vi "Collect and Set PWM.vi"(11 "Aircraft ID":u8) -> (3 "output cluster":T1)   [LabVIEW 2014]
uses:
  Aircraft Information/Sub VI/Get Aircraft RC Override.vi
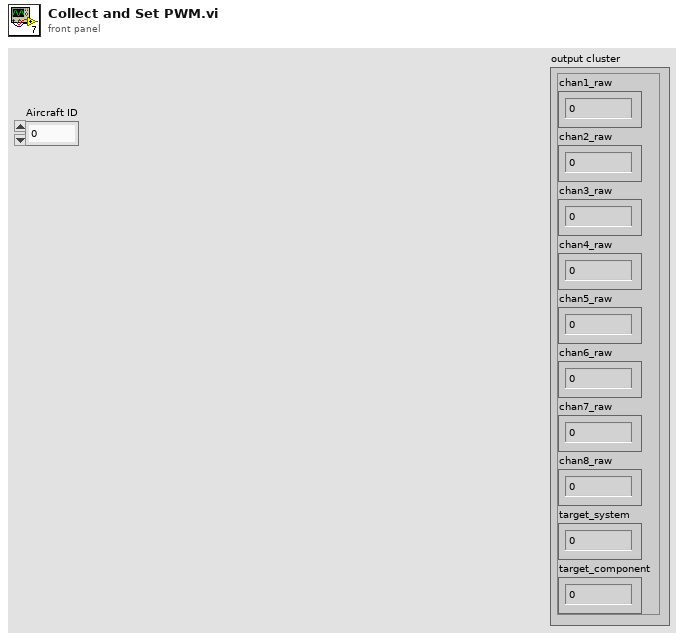
[diagram p1: front panel]
types:
  T1 = cluster{"chan1_raw":u16, "chan2_raw":u16, "chan3_raw":u16, "chan4_raw":u16, "chan5_raw":u16, "chan6_raw":u16, "chan7_raw":u16, "chan8_raw":u16, "target_system":u8, "target_component":u8}
  T2 = typedef "RC Override.ctl" = cluster{"Throttle":u16, "Roll":u16, "Pitch":u16, "Yaw":u16, "Arm":bool, "Disarm":bool, "Aircraft Mode":T3}
  T3 = typedef "Aircraft Mode.ctl" = enum16{"Loiter", "Stabalise", "Failsafe", "Emergency Stop"}
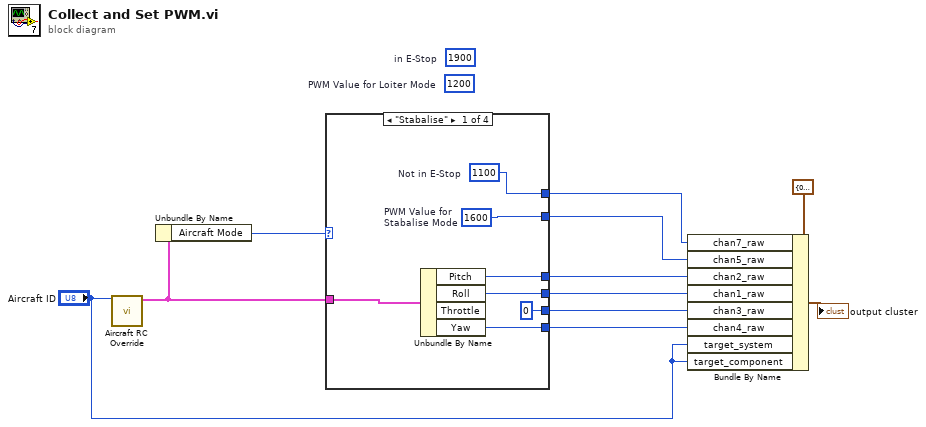
[diagram p0: block diagram]
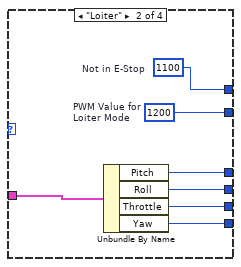
[diagram p2: hidden frame]
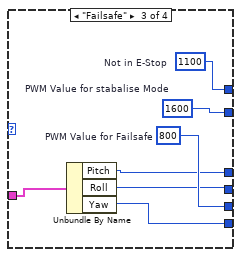
[diagram p3: hidden frame]
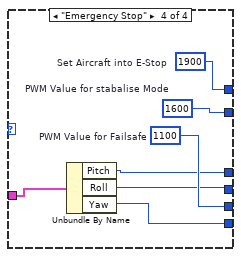
[diagram p4: hidden frame]
diagram:
  (unwired) u16 1900  # in E-Stop
  (unwired) u16 1200  # PWM Value for Loiter Mode
  n1 = call-poly "Aircraft RC Override.vi"("Aircraft ID"="Aircraft ID") -> ("RC Override Values Out"=w6:T2)  [unwired: 9 in, 1 out]
  n2 = Unbundle By Name(w6) -> ("Aircraft Mode"=w5:T3)
  n3 = case shown="\"Stabalise\"" w5 {
    tunnel: [w14 w21 w27 w34] -> w10
    tunnel: [w18 w25 w30 w37] -> w9
    tunnel: [w17 w24 w29 w36] -> w8
    tunnel: [w16 w23 w28 w35] -> w7
    tunnel: w6 -> [w15 w22 w31 w38]
    tunnel: [u16 0 ("PWM Value for Failsafe") w20 w32 w39] -> w4
    tunnel: [w12 w19 w26 w33] -> w1
    frame "Stabalise" {
      w12 = u16 1100  # Not in E-Stop
      w14 = u16 1600  # PWM Value for  Stabalise Mode
      n4 = Unbundle By Name(w15) -> ("Pitch"=w18:u16, "Roll"=w17:u16, "Yaw"=w16:u16)  [unwired: 1 out]
    }
    frame "Loiter" {
      w19 = u16 1100  # Not in E-Stop
      w21 = u16 1200  # PWM Value for  Loiter Mode
      n5 = Unbundle By Name(w22) -> ("Pitch"=w25:u16, "Roll"=w24:u16, "Throttle"=w20:u16, "Yaw"=w23:u16)
    }
    frame "Failsafe" {
      w26 = u16 1100  # Not in E-Stop
      w27 = u16 1600  # PWM Value for stabalise Mode
      w32 = u16 800  # PWM Value for Failsafe
      n6 = Unbundle By Name(w31) -> ("Pitch"=w30:u16, "Roll"=w29:u16, "Yaw"=w28:u16)
    }
    frame "Emergency Stop" {
      w33 = u16 1900  # Set Aircraft into E-Stop
      w34 = u16 1600  # PWM Value for stabalise Mode
      w39 = u16 1100  # PWM Value for Failsafe
      n7 = Unbundle By Name(w38) -> ("Pitch"=w37:u16, "Roll"=w36:u16, "Yaw"=w35:u16)
    }
  }
  n8 = Bundle By Name(cluster=T1 {"chan1_raw"=0, "chan2_raw"=0, "chan3_raw"=0, "chan4_raw"=0, "chan5_raw"=0, "chan6_raw"=0, "chan7_raw"=0, "chan8_raw"=0, "target_system"=0, "target_component"=0} ("Payload"), "chan7_raw"=w1, "chan5_raw"=w10, "chan2_raw"=w9, "chan1_raw"=w8, "chan3_raw"=w4, "chan4_raw"=w7, "target_system"="Aircraft ID", "target_component"="Aircraft ID") -> (→"output cluster":T1)
